vi "Set Ring Text.vi"(9 "Items":string[](array[string]), 11 "Rings":refnum<vi>[](array[refnum])) -> (0 "error out":errorcluster, 2 "data changed":bool)   [LabVIEW 2020, in "PXISlotGP.xctl"]
uses:
  PXISlotGP.xctl
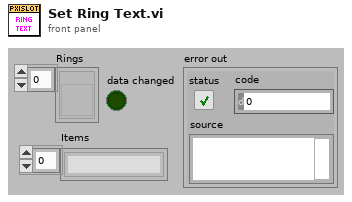
[diagram p1: front panel]
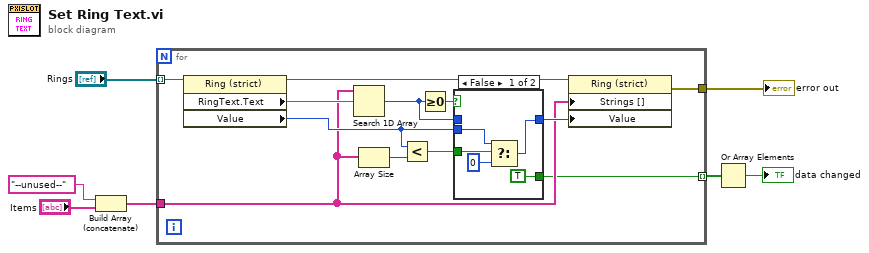
[diagram p0: block diagram]
diagram:
  n1 = Build Array (concatenate)("--unused--", "Items") -> (w4:string[])
  n2 = for {
    tunnel: "Rings" -> [w18] mode=indexing
    tunnel: w4 -> [w10]
    tunnel: [w19] -> w3
    tunnel: [w8] -> w2 mode=indexing
    n3 = property class="Ring (strict)"(reference=w18) -> (reference out=w17:refnum<vi>, "RingText.Text"=w16:string, "Value"=w12:u16)  [unwired: 1 in, 1 out]
    n4 = Search 1D Array(1D array=w10, element=w16) -> (index of element=w14:i32)  [unwired: 1 in]
    n5 = Array Size(array=w10) -> (size(s)=w11:i32)
    n6 = Less?(x=w12, y=w11) -> (x < y?=w9:bool)
    n7 = Greater Or Equal To 0?(x=w14) -> (x >= 0?=w15:bool)
    n8 = case shown="False" w15 {
      tunnel: w14 -> [_ w25]
      tunnel: [w21 w25] -> w13
      tunnel: w12 -> [w23 _]
      tunnel: w9 -> [w24 _]
      tunnel: [TRUE _] -> w8
      frame False {
        n9 = Select(t=w23, s=w24, f=u16 0) -> (s? t:f=w21:u16)
      }
      frame True {
      }
    }
    n10 = property class="Ring (strict)"(reference=w17, "Strings []"=w10, "Value"=w13) -> (error out=w19:errorcluster)  [unwired: 1 in, 1 out]
  }
  "error out" <- w3
  n11 = Or Array Elements(Boolean array=w2) -> (logical OR=→"data changed":bool)
